vi "Tryb SubVI.vi"(6 "error in":errorcluster, 8 "Drying":bool=TRUE, 9 "Lid":bool=TRUE, 10 "Czas":dbl, 11 "Enum":T2) -> (2 "output cluster":T1, 3 "End?":bool, 4 "error out":errorcluster)   [LabVIEW 2015]
uses:
  Controls/States.ctl
  Controls/Cluster.ctl
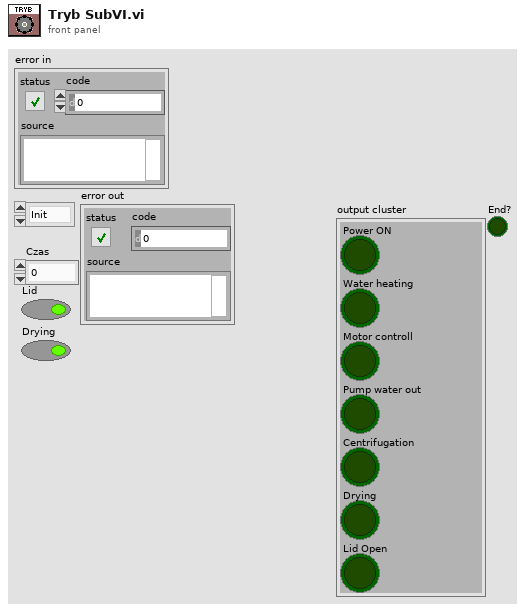
[diagram p1: front panel]
types:
  T1 = typedef "Cluster.ctl" = cluster{"Power ON":bool, "Water heating":bool, "Motor controll":bool, "Pump water out":bool, "Centrifugation":bool, "Drying":bool, "Lid Open":bool}
  T2 = typedef "States.ctl" = enum16{"Init", "Idle", "Cotton", "Silk", "Fast", "Drying"}
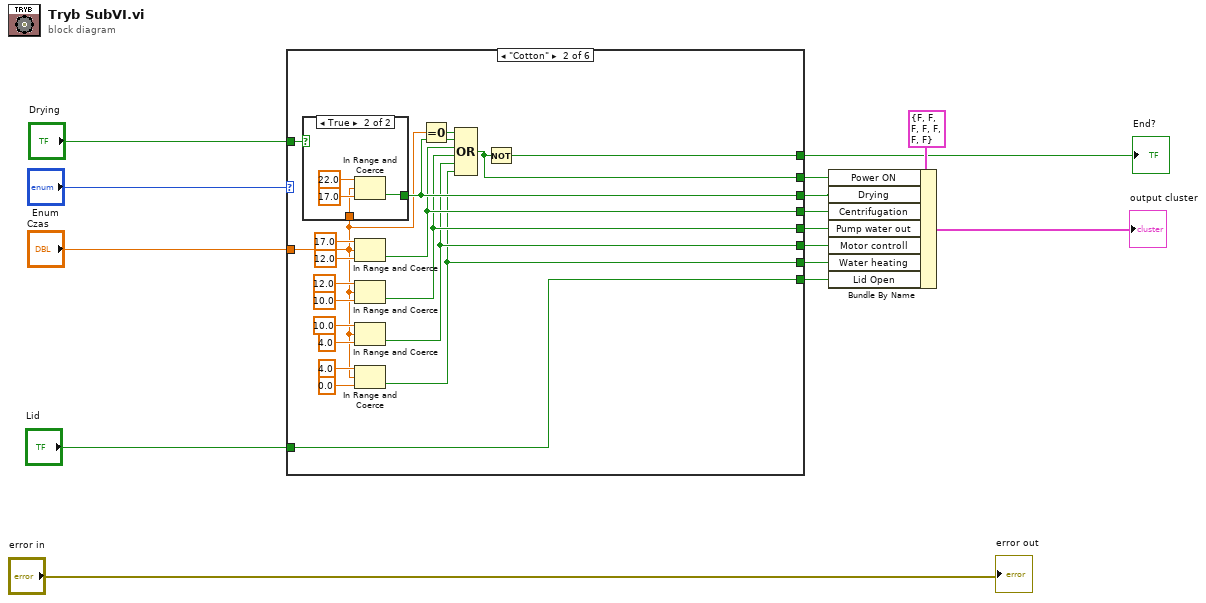
[diagram p0: block diagram]
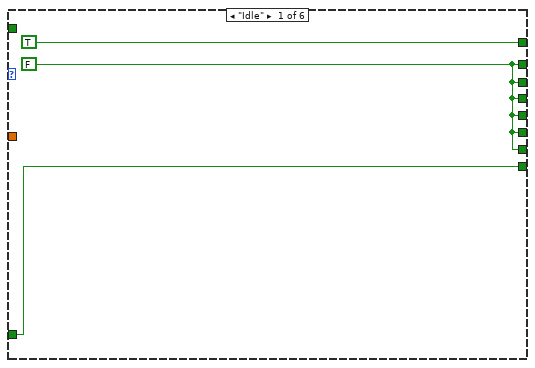
[diagram p2: hidden frame]
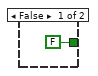
[diagram p3: hidden frame]
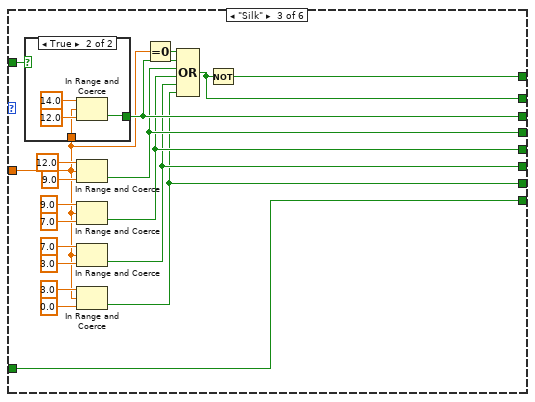
[diagram p4: hidden frame]
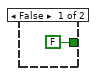
[diagram p5: hidden frame]
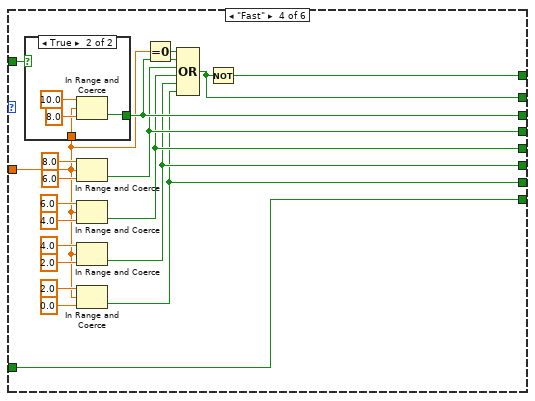
[diagram p6: hidden frame]
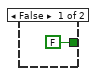
[diagram p7: hidden frame]
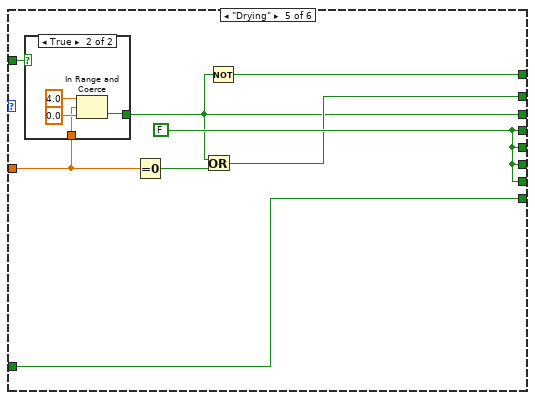
[diagram p8: hidden frame]
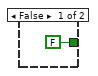
[diagram p9: hidden frame]
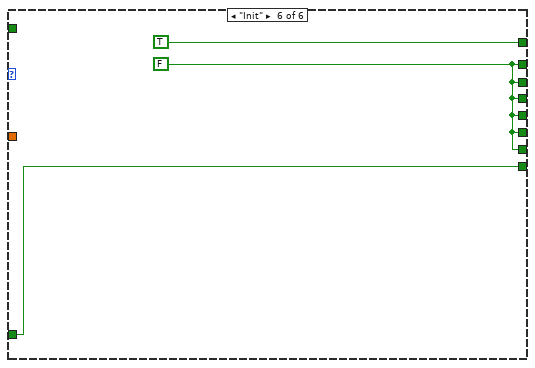
[diagram p10: hidden frame]
diagram:
  n1 = case shown="\"Cotton\"" "Enum" {
    tunnel: "Czas" -> [_ w19 w43 w67 w91 _]
    tunnel: "Drying" -> [_ w29 w53 w77 w98 _]
    tunnel: [TRUE w28 w52 w76 w97 TRUE] -> w7
    tunnel: "Lid" -> [w16 w21 w45 w69 w96 w104]
    tunnel: [w17 w27 w51 w75 w93 w105] -> w10
    tunnel: [w17 w26 w50 w74 w94 w105] -> w9
    tunnel: [w17 w25 w49 w73 w95 w105] -> w6
    tunnel: [w17 w24 w48 w72 w95 w105] -> w5
    tunnel: [w17 w23 w47 w71 w95 w105] -> w4
    tunnel: [w17 w22 w46 w70 w95 w105] -> w3
    tunnel: [w16 w21 w45 w69 w96 w104] -> w2
    frame "Idle" {
      w17 = FALSE
    }
    frame "Cotton" {
      n2 = case shown="True" w29 {
        tunnel: w19 -> [_ w40]
        tunnel: [FALSE w39] -> w27
        frame False {
        }
        frame True {
          n3 = In Range and Coerce(upper limit=22.0, x=w40, lower limit=17.0) -> (In Range?=w39:bool)  [unwired: 1 out]
        }
      }
      n4 = In Range and Coerce(upper limit=17.0, x=w19, lower limit=12.0) -> (In Range?=w25:bool)  [unwired: 1 out]
      n5 = In Range and Coerce(upper limit=12.0, x=w19, lower limit=10.0) -> (In Range?=w24:bool)  [unwired: 1 out]
      n6 = In Range and Coerce(upper limit=10.0, x=w19, lower limit=4.0) -> (In Range?=w23:bool)  [unwired: 1 out]
      n7 = In Range and Coerce(upper limit=4.0, x=w19, lower limit=0.0) -> (In Range?=w22:bool)  [unwired: 1 out]
      n8 = Equal To 0?(x=w19) -> (x = 0?=w20:bool)
      n9 = Compound Arithmetic op=OR(w20, w27, w25, w24, w23, w22) -> (w26:bool)
      n10 = Not(x=w26) -> (.not. x?=w28:bool)
    }
    frame "Silk" {
      n11 = case shown="True" w53 {
        tunnel: w43 -> [_ w64]
        tunnel: [FALSE w63] -> w51
        frame False {
        }
        frame True {
          n12 = In Range and Coerce(upper limit=14.0, x=w64, lower limit=12.0) -> (In Range?=w63:bool)  [unwired: 1 out]
        }
      }
      n13 = In Range and Coerce(upper limit=12.0, x=w43, lower limit=9.0) -> (In Range?=w49:bool)  [unwired: 1 out]
      n14 = In Range and Coerce(upper limit=9.0, x=w43, lower limit=7.0) -> (In Range?=w48:bool)  [unwired: 1 out]
      n15 = In Range and Coerce(upper limit=7.0, x=w43, lower limit=3.0) -> (In Range?=w47:bool)  [unwired: 1 out]
      n16 = In Range and Coerce(upper limit=3.0, x=w43, lower limit=0.0) -> (In Range?=w46:bool)  [unwired: 1 out]
      n17 = Equal To 0?(x=w43) -> (x = 0?=w44:bool)
      n18 = Compound Arithmetic op=OR(w44, w51, w49, w48, w47, w46) -> (w50:bool)
      n19 = Not(x=w50) -> (.not. x?=w52:bool)
    }
    frame "Fast" {
      n20 = case shown="True" w77 {
        tunnel: w67 -> [_ w88]
        tunnel: [FALSE w87] -> w75
        frame False {
        }
        frame True {
          n21 = In Range and Coerce(upper limit=10.0, x=w88, lower limit=8.0) -> (In Range?=w87:bool)  [unwired: 1 out]
        }
      }
      n22 = In Range and Coerce(upper limit=8.0, x=w67, lower limit=6.0) -> (In Range?=w73:bool)  [unwired: 1 out]
      n23 = In Range and Coerce(upper limit=6.0, x=w67, lower limit=4.0) -> (In Range?=w72:bool)  [unwired: 1 out]
      n24 = In Range and Coerce(upper limit=4.0, x=w67, lower limit=2.0) -> (In Range?=w71:bool)  [unwired: 1 out]
      n25 = In Range and Coerce(upper limit=2.0, x=w67, lower limit=0.0) -> (In Range?=w70:bool)  [unwired: 1 out]
      n26 = Equal To 0?(x=w67) -> (x = 0?=w68:bool)
      n27 = Compound Arithmetic op=OR(w68, w75, w73, w72, w71, w70) -> (w74:bool)
      n28 = Not(x=w74) -> (.not. x?=w76:bool)
    }
    frame "Drying" {
      w95 = FALSE
      n29 = case shown="True" w98 {
        tunnel: w91 -> [_ w101]
        tunnel: [FALSE w100] -> w93
        frame False {
        }
        frame True {
          n30 = In Range and Coerce(upper limit=4.0, x=w101, lower limit=0.0) -> (In Range?=w100:bool)  [unwired: 1 out]
        }
      }
      n31 = Equal To 0?(x=w91) -> (x = 0?=w92:bool)
      n32 = Or(x=w93, y=w92) -> (x .or. y?=w94:bool)
      n33 = Not(x=w93) -> (.not. x?=w97:bool)
    }
    frame "Init" {
      w105 = FALSE
    }
  }
  "End?" <- w7
  n34 = Bundle By Name(cluster=T1 {"Power ON"=FALSE, "Water heating"=FALSE, "Motor controll"=FALSE, "Pump water out"=FALSE, "Centrifugation"=FALSE, "Drying"=FALSE, "Lid Open"=FALSE} ("Cluster 2"), "Power ON"=w9, "Drying"=w10, "Centrifugation"=w6, "Pump water out"=w5, "Motor controll"=w4, "Water heating"=w3, "Lid Open"=w2) -> (→"output cluster":T1)
  "error out" <- "error in"
